vi "GlobalVar.vi"() -> ()   [LabVIEW 2011]
panel:
  in  "T rate [K/min]":dbl=0.1 min=-200.0 max=200.0
  in  "Stabilization Time (s)":i32 min=-200 max=200
  in  "Conversion Factor VI 4\n1 V = ??":dbl=1.0
  in  "Conversion Factor IOL ramp\n1 V = ??":dbl=1.0
  out "Fix type":string
  out "Sweep type":string
  out "Stabilizing":bool=TRUE
  in  "PEM present ?":bool=TRUE
  in  "PEM VISA":refnum<visa-resource-name>
  in  "LaserControl":T1={"Power Stabilization"=TRUE, "Laser Power [W]"=0.0, "Power precision"=0.05} {"Laser Power [W]" format="%#.2g"}
  in  "Set Persistent":bool=TRUE
  in  "V step [V]":dbl=0.001
  in  "Sweep rate [T/min]":dbl=0.1 min=-200.0 max=200.0
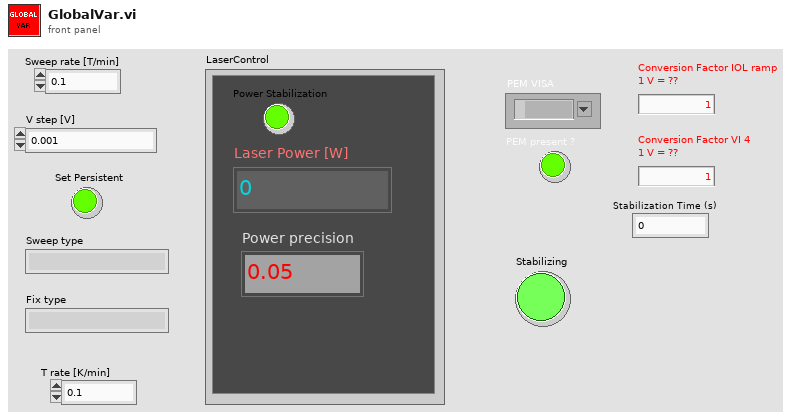
[diagram p1: front panel]
types:
  T1 = cluster{"Power Stabilization":bool, "Laser Power [W]":dbl, "Power precision":dbl}
diagram:
